vi "75_Vision_RC Servo_DC_Moto_test_PID.vi"() -> ()   [LabVIEW 2018]
uses:
  <userlib>/KNR OS 4.0 LabVIEW Toolkit/Type Definition/Resource.ctl
  <userlib>/KNR OS 4.0 LabVIEW Toolkit/Type Definition/RC Servo Port.ctl
  <userlib>/KNR OS 4.0 LabVIEW Toolkit/Type Definition/DC Motor Port.ctl
panel:
  out "RS2":dbl
  out "RS1":dbl
  out "LS2":dbl
  out "LS1":dbl
  out "VR":dbl
  out "VL":dbl
  out "Waveform Chart":dbl(graph)
  in  "Kd":dbl(slide)=0.06 scale=0.0..0.1
  in  "Ki":dbl(slide)=0.025 scale=0.0..0.1
  in  "Kp":dbl(slide)=0.05 scale=0.0..0.2
  out "area":dbl
  out "RC Pulse Width (uS)":u16[](array[numeric])
  out "Image Out":T1(plugin-control)
  in  "stop":bool
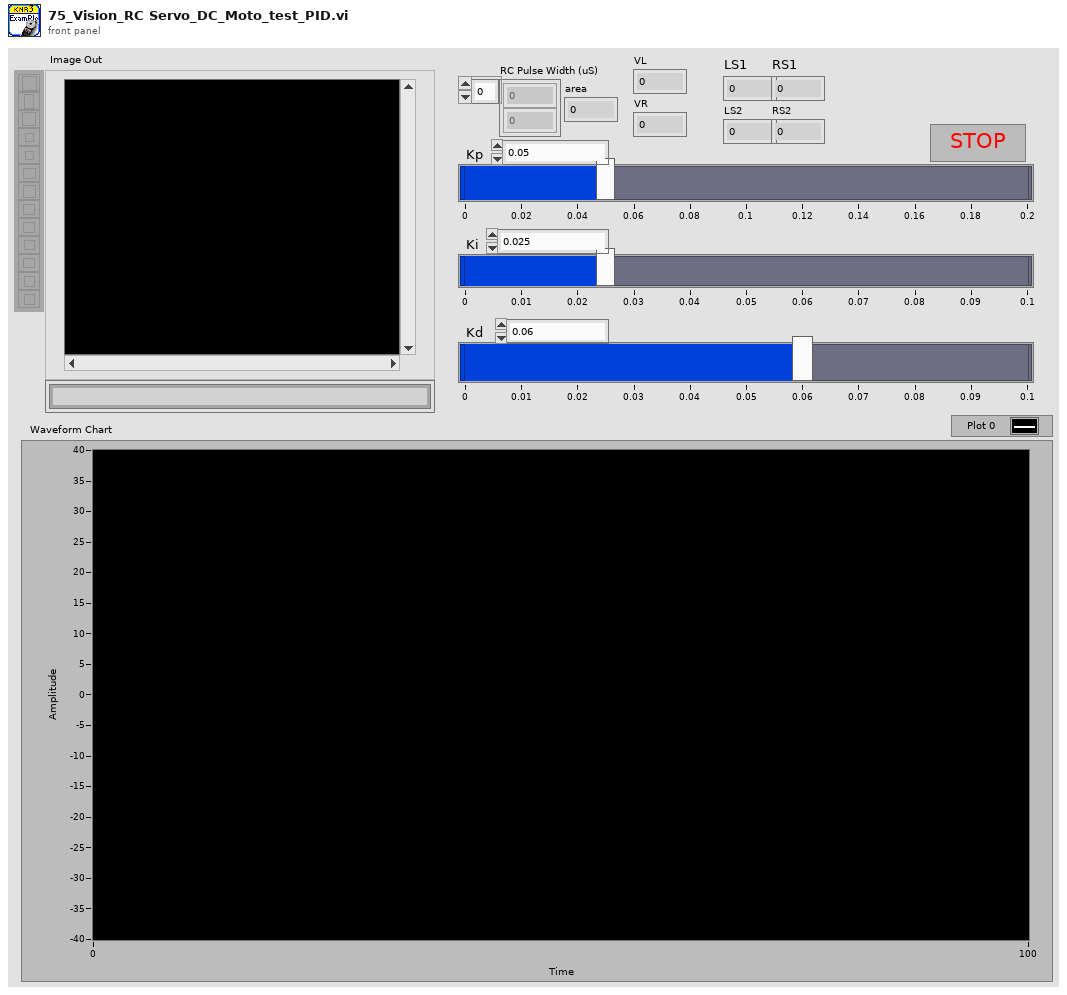
[diagram p1: front panel]
types:
  T1 = typedef "IMAQ Image.ctl" = refnum<image>
  T2 = typedef "DC Motor Port.ctl" = u16
  T3 = typedef "RC Servo Port.ctl" = u16
  T4 = typedef "Resource.ctl" = enum16{"KNRm_DDRC", "KNRm_DDDD", "KNRm_DDDR", "KNRm_DDDC", "KNR", "KNRm_neww"}
  T5 = typedef "KNR3 Reference.ctl" = cluster{"FPGA Session":refnum<class "FPGA Interface Base.lvclass">, "Resource":T4}
  T6 = cluster{"Left":dbl, "Top":dbl, "Right":dbl, "Bottom":dbl}
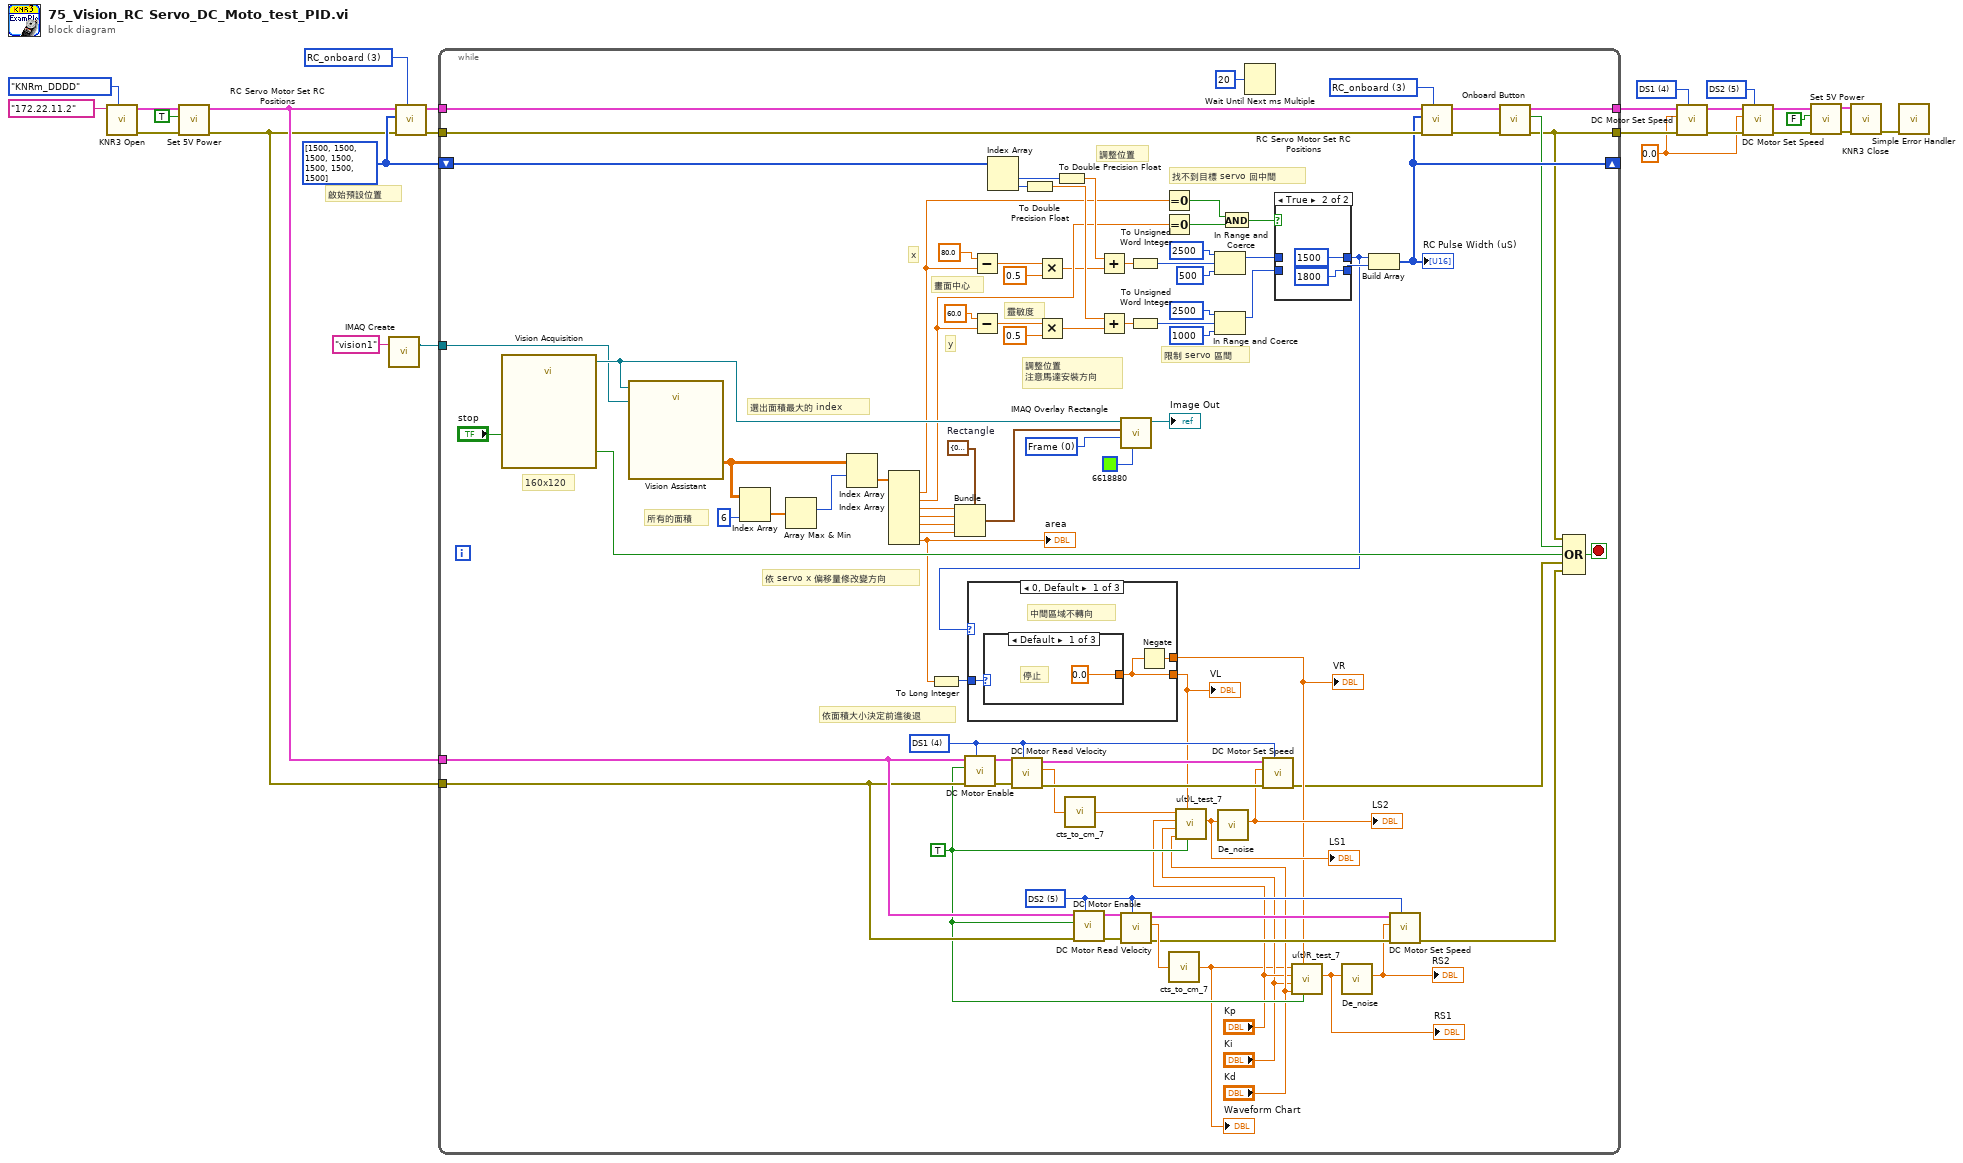
[diagram p0: block diagram]
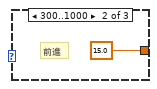
[diagram p2: hidden frame]
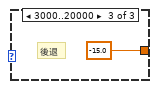
[diagram p3: hidden frame]
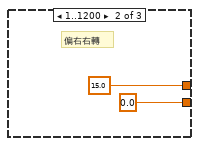
[diagram p4: hidden frame]
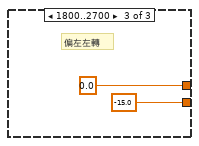
[diagram p5: hidden frame]
diagram:
  w1 = T2 5 items=["DS1"=4, "DS2"=5, "DS3"=6, "DS4"=7] ("Port (DS1)")
  w2 = T2 4 items=["DS1"=4, "DS2"=5, "DS3"=6, "DS4"=7] ("Port (DS1)")
  w3 = 0.0 ("Speed (+-100%)")
  w13 = u16[] [1500, 1500, 1500, 1500, 1500, 1500, 1500] ("RC Pulse Width (1500 uS)")
  w16 = T3 3 items=["RC_onboard"=3, "RC_box"=9] ("Port (RC_onboard)")
  # "啟始預設位置"
  n1 = call <userlib>:"KNR3 Open.vi"("Resource"=Resource."KNRm_DDDD", "IP"="172.22.11.2") -> ("error out"=w22:errorcluster, "KNR out"=w23:T5)  [unwired: 8 in]
  n2 = call <userlib>:"Set 5V Power.vi"("error in (no error)"=w22, "5V Power(T)"=TRUE ("5V Power"), "KNR in"=w23) -> ("error out"=w11:errorcluster, "KNR out"=w12:T5)  [unwired: 7 in]
  n3 = call "IMAQ Create"("Image Name"="vision1") -> ("New Image"=w14:T1)  [unwired: 4 in, 1 out]
  n4 = call <userlib>:"RC Servo Motor Set RC Positions.vi"("Port (RC_onboard)"=w16, "RC Pulse Width (1500 uS)"=w13, "KNR in"=w12) -> ("KNR out"=w17:T5)  [unwired: 7 in, 1 out]
  n5 = while {
    tunnel: w17 -> [w111]
    tunnel: [w40] -> w10
    tunnel: w11 -> [w109]
    tunnel: [w38] -> w9
    tunnel: w14 -> [w91]
    shift-right: [w75] -> _
    shift-left: w13 -> [w78]
    tunnel: w12 -> [w45]
    tunnel: w11 -> [w44]
    stop <- w108 stop-if-true
    w43 = u32 0 items=["Frame", "Fill", "Highlight"] ("Drawing Mode (Frame)")
    w47 = T2 5 items=["DS1"=4, "DS2"=5, "DS3"=6, "DS4"=7] ("Port 2")
    w41 = TRUE ("Enable Motor(F)")
    w59 = T2 4 items=["DS1"=4, "DS2"=5, "DS3"=6, "DS4"=7] ("Port 2")
    w104 = T6 {"Left"=0.0, "Top"=0.0, "Right"=0.0, "Bottom"=0.0}  # Rectangle
    w106 = T3 3 items=["RC_onboard"=3, "RC_box"=9] ("RC Motor")
    # "調整位置\n注意馬達安裝方向"
    # "依面積大小決定前進後退"
    # "依 servo x 偏移量修改變方向"
    # "調整位置"
    # "靈敏度"
    # "所有的面積"
    # "畫面中心"
    # "限制 servo 區間"
    # "找不到目標 servo 回中間"
    # "y"
    # "x"
    # "160x120"
    # "選出面積最大的 index"
    n6 = call "Vision Acquisition"("Stop (F)"="stop") -> ("Image Out"=w96:T1, "Stopped"=w89:bool)  [unwired: 24 in, 1 out]
    n7 = call "Vision Assistant"("Image In"=w96, "Image Dst"=w91) -> ("Particle Measurements (Pixels) (Particle Analysis 1)"=w95:dbl[][])  [unwired: 22 in, 3 out]
    n8 = Index Array "Index Array"(array=w95, index (col)=6 ("disabled index (col)")) -> (element=w94:dbl[])  [unwired: 1 in]
    n9 = Array Max & Min(array=w94) -> (max index (indices)=w93:i32)  [unwired: 3 out]
    n10 = Index Array "Index Array"(array=w95, index (row)=w93) -> (element=w105:dbl[])  [unwired: 1 in]
    n11 = Index Array "Index Array"(array=w105) -> (element #1=w68:dbl, element #2=w67:dbl, element #3=w103:dbl, element #4=w102:dbl, element #5=w101:dbl, element #6=w100:dbl, element #7=w53:dbl)  [unwired: 7 in]
    "area" <- w53
    n12 = To Long Integer(number=w53) -> (32bit integer=w33:i32)
    n13 = Bundle "Bundle"(cluster=w104, "Left"=w103, "Top"=w102, "Right"=w101, "Bottom"=w100) -> (w99:T6)
    n14 = call <userlib>:"DC Motor Enable.vi"("Port (DS1)"=w59, "error in (no error)"=w44, "Enable Motor(F)"=w41, "KNR in"=w45) -> ("error out"=w55:errorcluster, "KNR out"=w54:T5)  [unwired: 6 in]
    n15 = Subtract(x=80.0 ("y"), y=w68) -> (x-y=w85:dbl)
    n16 = Subtract(x=60.0 ("y"), y=w67) -> (x-y=w86:dbl)
    n17 = Index Array "Index Array"(array=w78) -> (element #1=w77:u16, element #2=w76:u16)  [unwired: 2 in]
    n18 = call <userlib>:"DC Motor Read Velocity.vi"("Port (DS1)"=w59, "error in (no error)"=w55, "KNR in"=w54) -> ("error out"=w58:errorcluster, "Velocity (cts/sec)"=w56:dbl, "KNR out"=w57:T5)  [unwired: 6 in]
    n19 = To Double Precision Float(number=w76) -> (double precision float=w69:dbl)
    n20 = Multiply(x=w85, y=0.5) -> (x*y=w66:dbl)
    n21 = Multiply(x=w86, y=0.5) -> (x*y=w65:dbl)
    n22 = To Double Precision Float(number=w77) -> (double precision float=w70:dbl)
    n23 = call "cts_to_cm_7.vi"("cts"=w56) -> ("cm"=w42:dbl)
    n24 = call <userlib>:"DC Motor Enable.vi"("Port (DS1)"=w47, "error in (no error)"=w44, "Enable Motor(F)"=w41, "KNR in"=w45) -> ("error out"=w51:errorcluster, "KNR out"=w52:T5)  [unwired: 6 in]
    n25 = Add(x=w70, y=w66) -> (x+y=w87:dbl)
    n26 = Add(x=w69, y=w65) -> (x+y=w88:dbl)
    n27 = call "IMAQ Overlay Rectangle"("Color"=u32 6618880, "Drawing Mode (Frame)"=w43, "Rectangle"=w99, "Image"=w96) -> ("Image Out"=→"Image Out":T1)  [unwired: 6 in, 1 out]
    n28 = call <userlib>:"DC Motor Read Velocity.vi"("Port (DS1)"=w47, "error in (no error)"=w51, "KNR in"=w52) -> ("error out"=w48:errorcluster, "Velocity (cts/sec)"=w50:dbl, "KNR out"=w49:T5)  [unwired: 6 in]
    n29 = To Unsigned Word Integer(number=w87) -> (unsigned 16bit integer=w72:u16)
    n30 = To Unsigned Word Integer(number=w88) -> (unsigned 16bit integer=w71:u16)
    n31 = Equal To 0?(x=w68) -> (x = 0?=w63:bool)
    n32 = Equal To 0?(x=w67) -> (x = 0?=w64:bool)
    n33 = call "cts_to_cm_7.vi"("cts"=w50) -> ("cm"=w25:dbl)
    "Waveform Chart" <- w25
    n34 = In Range and Coerce(upper limit=u16 2500, x=w72, lower limit=u16 500) -> (coerced(x)=w62:u16)  [unwired: 1 out]
    n35 = In Range and Coerce(upper limit=u16 2500, x=w71, lower limit=u16 1000) -> (coerced(x)=w61:u16)  [unwired: 1 out]
    n36 = And(x=w63, y=w64) -> (x .and. y?=w29:bool)
    n37 = Wait Until Next ms Multiple(millisecond multiple=u32 20) -> ()  [unwired: 1 out]
    n38 = case shown="True" w29 {
      tunnel: w62 -> [w123 _]
      tunnel: w61 -> [w122 _]
      tunnel: [w123 u16 1500] -> w34
      tunnel: [w122 u16 1800] -> w60
      frame False {
      }
      frame True {
      }
    }
    n39 = case shown="0, Default" w34 {
      tunnel: [w113 0.0 -15.0] -> w32
      tunnel: [w114 15.0 0.0] -> w31
      tunnel: w33 -> [w112 _ _]
      frame 0, Default {
        # "中間區域不轉向"
        n40 = case shown="Default" w112 {
          tunnel: [0.0 15.0 -15.0] -> w113
          frame Default {
            # "停止"
          }
          frame 300..1000 {
            # "前進"
          }
          frame 3000..20000 {
            # "後退"
          }
        }
        n41 = Negate(x=w113) -> (-x=w114:dbl)
      }
      frame 1..1200 {
        # "偏右右轉"
      }
      frame 1800..2700 {
        # "偏左左轉"
      }
    }
    "VL" <- w32
    "VR" <- w31
    n42 = call "u(t)L_test_7.vi"("enable"=w41, "Desire Velosity"=w32, "Kd"="Kd", "Ki"="Ki", "Kp"="Kp", "Velocity"=w42) -> ("u(t)"=w36:dbl)  [unwired: 5 in]
    "LS1" <- w36
    n43 = call "De_noise.vi"("u(t)"=w36) -> ("u(t)2"=w37:dbl)  [unwired: 6 in]
    "LS2" <- w37
    n44 = call <userlib>:"DC Motor Set Speed.vi"("Port (DS1)"=w59, "error in (no error)"=w58, "Speed (+-100%)"=w37, "KNR in"=w57) -> ("error out"=w30:errorcluster)  [unwired: 6 in, 1 out]
    n45 = call "u(t)R_test_7.vi"("enable"=w41, "Desire Velosity"=w31, "Kd"="Kd", "Ki"="Ki", "Kp"="Kp", "Velocity"=w25) -> ("u(t)"=w24:dbl)  [unwired: 5 in]
    "RS1" <- w24
    n46 = call "De_noise.vi"("u(t)"=w24) -> ("u(t)2"=w35:dbl)  [unwired: 6 in]
    "RS2" <- w35
    n47 = Build Array "Build Array"(w34, w60) -> (w75:u16[])
    "RC Pulse Width (uS)" <- w75
    n48 = call <userlib>:"DC Motor Set Speed.vi"("Port (DS1)"=w47, "error in (no error)"=w48, "Speed (+-100%)"=w35, "KNR in"=w49) -> ("error out"=w46:errorcluster)  [unwired: 6 in, 1 out]
    n49 = call <userlib>:"RC Servo Motor Set RC Positions.vi"("Port (RC_onboard)"=w106, "error in (no error)"=w109, "RC Pulse Width (1500 uS)"=w75, "KNR in"=w111) -> ("error out"=w38:errorcluster, "KNR out"=w110:T5)  [unwired: 6 in]
    n50 = call <userlib>:"Onboard Button.vi"("KNR in"=w110) -> ("value"=w39:bool, "KNR out"=w40:T5)  [unwired: 8 in, 1 out]
    n51 = Compound Arithmetic op=OR(w38, w39, w89, w30, w46) -> (w108:bool)
  }
  n52 = call <userlib>:"DC Motor Set Speed.vi"("Port (DS1)"=w2, "Speed (+-100%)"=w3, "KNR in"=w10) -> ("KNR out"=w5:T5)  [unwired: 7 in, 1 out]
  n53 = call <userlib>:"DC Motor Set Speed.vi"("Port (DS1)"=w1, "Speed (+-100%)"=w3, "KNR in"=w5) -> ("KNR out"=w4:T5)  [unwired: 7 in, 1 out]
  n54 = call <userlib>:"Set 5V Power.vi"("error in (no error)"=w9, "5V Power(T)"=FALSE, "KNR in"=w4) -> ("error out"=w7:errorcluster, "KNR out"=w8:T5)  [unwired: 7 in]
  n55 = call <userlib>:"KNR3 Close.vi"("error in (no error)"=w7, "KNR in"=w8) -> ("error out"=w21:errorcluster)  [unwired: 9 in]
  n56 = call <vilib>:"Simple Error Handler.vi"("error in (no error)"=w21) -> ()  [unwired: 4 in, 5 out]
